vi "Untitled 612.vi"() -> ()   [LabVIEW 2009]
panel:
  out "unsigned byte array 2":u8[](array[numeric])
  out "ASCII string":string
  in  "string 3":string
  out "number":u32
  out "hex integer string":string
  in  "1st stage":u8[](array[numeric])=[0, 0, 0, 0, 0, 0, 0, 0, 0, 0]
  out "string 2":string
  out "unsigned byte array":u8[](array[numeric])
  in  "string":string
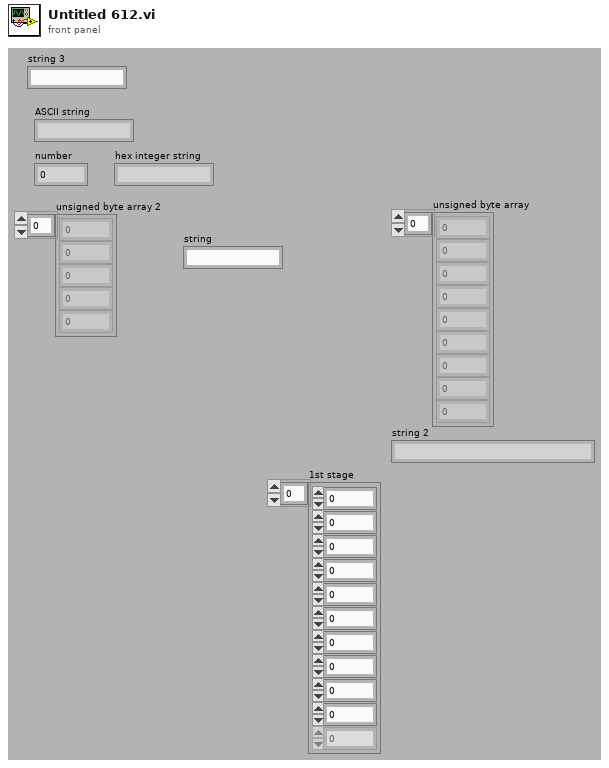
[diagram p1: front panel]
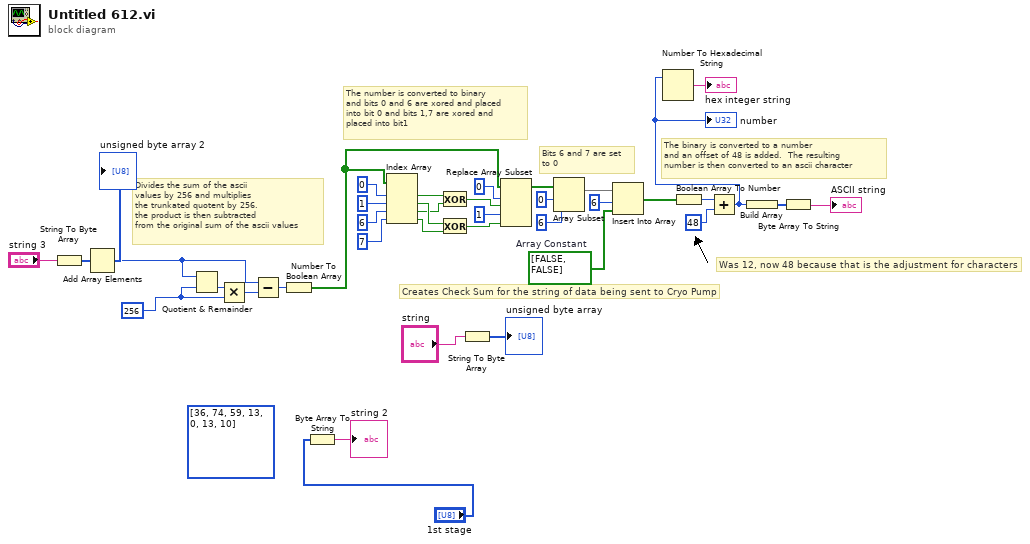
[diagram p0: block diagram]
diagram:
  w25 = bool[] [FALSE, FALSE]  # Array Constant
  w2 = 256 ("y")
  (unwired) u8[] [36, 74, 59, 13, 0, 13, 10] ("unsigned byte array")
  # "Was 12, now 48 because that is the adjustment for characters"
  # "The binary is converted to a number\nand an offset of 48 is added.  The resulting\nnumber is then converted to an ascii character"
  # "Bits 6 and 7 are set\nto 0"
  # "The number is converted to binary\nand bits 0 and 6 are xored and placed\ninto bit 0 and bits 1,7 are xored and\nplaced into bit1"
  # "Divides the sum of the ascii\nvalues by 256 and multiplies\nthe trunkated quotent by 256.\nthe product is then subtracted\nfrom the original sum of the ascii values"
  # "Creates Check Sum for the string of data being sent to Cryo Pump"
  n1 = String To Byte Array(string="string 3") -> (unsigned byte array=w20:u8[])
  "unsigned byte array 2" <- w20
  n2 = Add Array Elements(numeric array=w20) -> (sum=w19:u8)
  n3 = Quotient & Remainder(x=w19, y=w2) -> (floor(x/y)=w3:i32)  [unwired: 1 out]
  n4 = Multiply(x=w3, y=w2) -> (x*y=w1:i32)
  n5 = Subtract(x=w19, y=w1) -> (x-y=w4:i32)
  n6 = Number To Boolean Array(number=w4) -> (Boolean array=w14:bool[])
  n7 = Byte Array To String(unsigned byte array="1st stage") -> (string=→"string 2":string)
  n8 = Index Array(array=w14, index #1=0 ("Index"), index #2=1 ("Index"), index #3=6 ("Index"), index #4=7 ("Index")) -> (element #1=w9:bool, element #2=w11:bool, element #3=w10:bool, element #4=w12:bool)
  n9 = Exclusive Or(1:w10, 2:w9) -> (0:w16:bool)
  n10 = Exclusive Or(1:w12, 2:w11) -> (0:w17:bool)
  n11 = String To Byte Array(string="string") -> (unsigned byte array=→"unsigned byte array":u8[])
  n12 = Replace Array Subset(array=w14, new element #1=w16, index #1=0 ("Index"), new element #2=w17, index #2=1 ("Index")) -> (w27:bool[])
  n13 = Array Subset(array=w27, index=0 ("Array Index"), length=6 ("Array Length")) -> (w28:bool[])
  n14 = Insert Into Array(array=w28, index=6 ("Index"), new element=w25) -> (w26:bool[])
  n15 = Boolean Array To Number(Boolean array=w26) -> (number=w31:u32)
  n16 = Add(x=w31, y=u32 48) -> (x+y=w33:u32)
  "number" <- w33
  n17 = Number To Hexadecimal String(2:w33) -> (0:→"hex integer string":string)  [unwired: 1 in]
  n18 = Build Array(w33) -> (w22:u32[])
  n19 = Byte Array To String(unsigned byte array=w22) -> (string=→"ASCII string":string)
